vi "ElevFF_MinAchieveAccel.vi"(9 "Velocity":dbl, 10 "MaxVoltage":dbl, 11 "in ELEV_FF":T1 {"Kg" format="%13.5p"; "Ka" format="%13.5p"; "Kv" format="%13.5p"; "Ks" format="%13.5p"}) -> (3 "MinAccel":dbl)   [LabVIEW 2019, in "Trajectory_Library.lvlib"]
doc: "Calculates the minimum achievable acceleration given a maximum voltage supply and a velocity. Useful for ensuring that velocity and acceleration constraints for a trapezoidal profile are simultaneously achievable - enter the velocity constraint, and this will give you a simultaneously-achievable acceleration constraint.\n \nInputs: \n - ElevFF -- The ElevFF data cluster\n - maxVoltage -- The maximum voltage that can be supplied to the elevator.\n - velocity -- The velocity of the elevator.\n\nOutputs:\n - MinAccel -- The minimum possible acceleration at the given velocity."
uses:
  Trajectory_Library.lvlib
  TypeDef/ELEV_FF.ctl
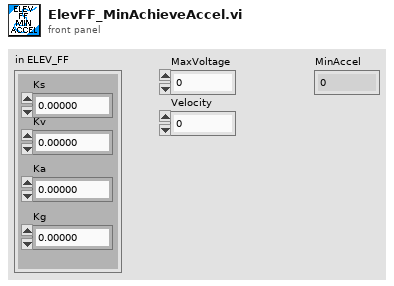
[diagram p1: front panel]
types:
  T1 = typedef "Trajectory_Library.lvlib/ELEV_FF.ctl" = cluster{"Ks":dbl, "Kv":dbl, "Ka":dbl, "Kg":dbl}
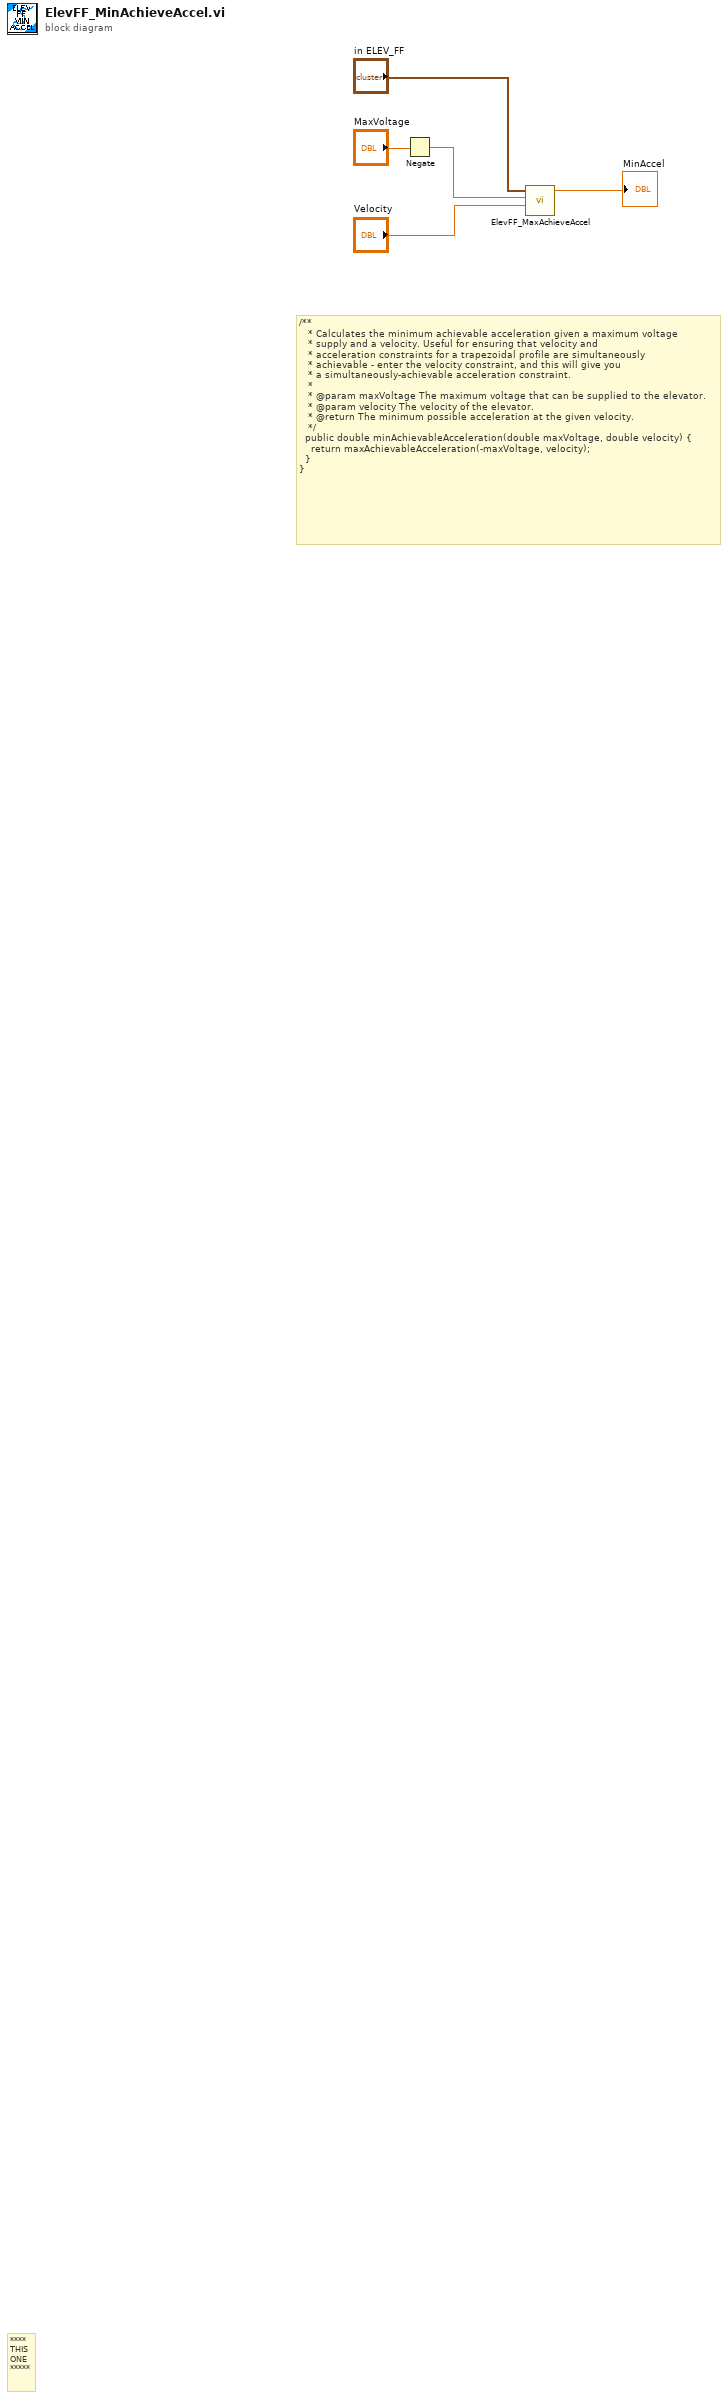
[diagram p0: block diagram]
diagram:
  # "/**\n   * Calculates the minimum achievable acceleration given a maximum voltage\n   * supply and a velocity. Useful for ensuring that velocity and\n   * acceleration constraints for a trapezoidal profile are simultaneously\n   * achievable - enter the velocity constraint, and this will give you\n   * a simultaneously-achievable acceleration constraint.\n   *\n   * @param maxVoltage The maximum voltage that can be supplied to the elevator.\n   * @param velocity The velocity of the elevator.\n   * @return The minimum possible acceleration at the given velocity.\n   */\n  public double minAchievableAcceleration(double maxVoltage, double velocity) {\n    return maxAchievableAcceleration(-maxVoltage, velocity);\n  }\n}"
  # "****\nTHIS\nONE\n*****"
  n1 = Negate(x="MaxVoltage") -> (-x=w3:dbl)
  n2 = call "ElevFF_MaxAchieveAccel.vi"("Velocity"="Velocity", "MaxVoltage"=w3, "in ELEV_FF"="in ELEV_FF") -> ("MaxAccel"=→"MinAccel":dbl)  [unwired: 8 in]
